vi "API.vi"() -> ()   [LabVIEW 2018]
uses:
  <vilib>/NI Veristand/Execution/Project/NI_VS Project ExecutionAPI.lvlib
  <vilib>/NI Veristand/Execution/Workspace/NI_VS Workspace ExecutionAPI.lvlib
  <vilib>/NI Veristand/Execution/ModelManager/NI_VS ModelManager ExecutionAPI.lvlib
  <vilib>/NI Veristand/Execution/Workspace/NI VeriStand - Get Multiple Channel Values.vi
  <vilib>/NI Veristand/Execution/ModelManager/NI VeriStand - Get Multiple Parameter Values.vi
  <vilib>/NI Veristand/Execution/ModelManager/NI VeriStand - Set Multiple Parameter Values.vi
  <vilib>/NI Veristand/Execution/DataLogging/NI_VS Data Logging API.lvlib
  <vilib>/NI Veristand/Execution/DataLogging/New Data Logging Specification (Text).vi
  <vilib>/NI Veristand/Execution/DataLogging/Text Channel.ctl
panel:
  in  "Channel Paths":T1[](array[typedef])
  in  "Session Name in":string="datalog"
  in  "Zapsat":bool
  out "Parametrz view":dbl[](array[numeric])
  in  "Parametry SET":dbl[](array[numeric])
  out "Aliases":string[](array[string])
  out "Parameters":string[](array[string])
  out "Values":dbl[](array[numeric])
  out "error out":errorcluster
  out "Channels":string[](array[string])
  in  "Project File Path":path=path "C:/Users/Public/Documents/National Instruments/NI VeriStand 2018/Projects/Example/Sinewave Delay.nivsproj"
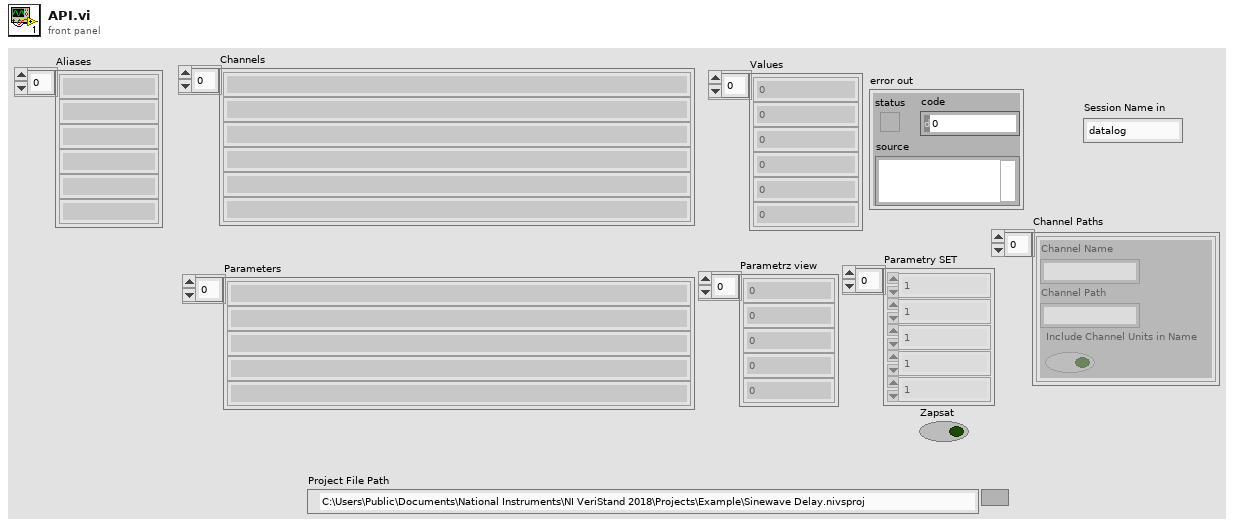
[diagram p1: front panel]
types:
  T1 = typedef "NI_VS Data Logging API.lvlib/Text Channel.ctl" = cluster{"Channel Name":string, "Channel Path":string, "Include Channel Units in Name":bool}
  T2 = typedef "NI_VS Project ExecutionAPI.lvlib/Project Ref.ctl" = refnum<k24>
  T3 = typedef "NI_VS Workspace ExecutionAPI.lvlib/WorkspaceAPI.ctl" = refnum<k24>
  T4 = typedef "NI_VS ModelManager ExecutionAPI.lvlib/ModelManagerAPI.ctl" = refnum<k24>
  T5 = typedef "NI_VS Data Logging API.lvlib/DataLoggingSpecification Ref.ctl" = refnum<k24>
  T6 = typedef "NI_VS Data Logging API.lvlib/IDataLogging Ref.ctl" = refnum<k24>
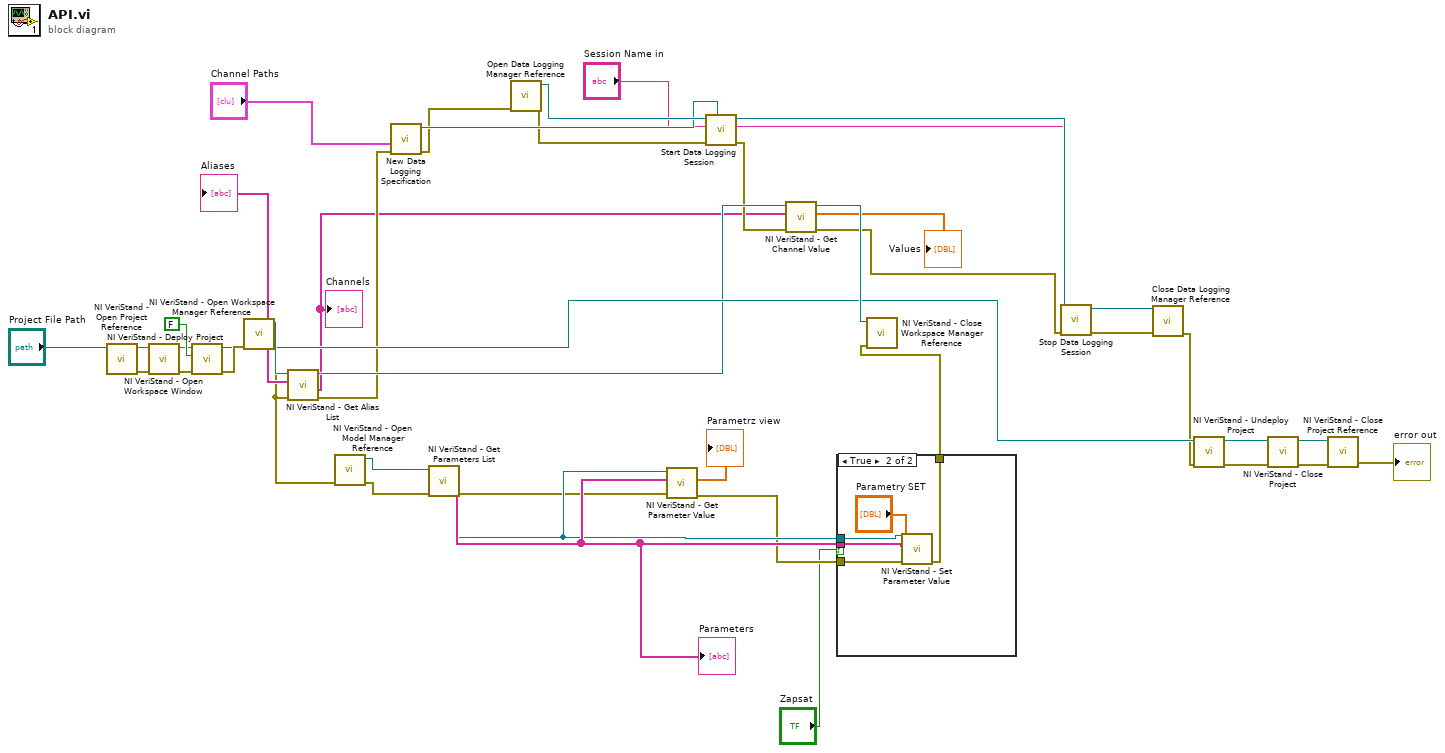
[diagram p0: block diagram]
diagram:
  n1 = call <vilib>:"NI VeriStand - Open Project Reference.vi"("Project File Path"="Project File Path") -> ("error out"=w40:errorcluster, "Project Ref"=w43:T2)  [unwired: 9 in]
  n2 = call <vilib>:"NI VeriStand - Open Workspace Window.vi"("error in (no error)"=w40, "Project Ref in"=w43) -> ("error out"=w39:errorcluster, "Project Ref out"=w35:T2)  [unwired: 8 in]
  n3 = call <vilib>:"NI VeriStand - Deploy Project.vi"("error in (no error)"=w39, "Show Progress (F)"=FALSE, "Project Ref in"=w35) -> ("error out"=w38:errorcluster, "Project Ref out"=w29:T2)  [unwired: 7 in]
  n4 = call <vilib>:"NI VeriStand - Open Workspace Manager Reference.vi"("error in (no error)"=w38) -> ("error out"=w23:errorcluster, "WorkspaceManager"=w36:T3)  [unwired: 9 in]
  n5 = call <vilib>:"NI VeriStand - Get Alias List.vi"("error in (no error)"=w23, "WorkspaceManager in"=w36) -> ("error out"=w7:errorcluster, "Channels"=w2:string[], "Aliases"=→"Aliases":string[], "WorkspaceManager out"=w27:T3)  [unwired: 6 in]
  "Channels" <- w2
  n6 = call <vilib>:"NI VeriStand - Open Model Manager Reference.vi"("error in (no error)"=w23) -> ("error out"=w24:errorcluster, "ModelManager"=w26:T4)  [unwired: 9 in]
  n7 = call-poly <vilib>:"New Data Logging Specification.vi"("error in (no error)"=w7, "Channel Paths"="Channel Paths") -> ("error out"=w6:errorcluster, "Data Logging Specification Ref out"=w12:T5)  [unwired: 8 in]
  n8 = call <vilib>:"NI VeriStand - Get Parameters List.vi"("error in (no error)"=w24, "ModelManager in"=w26) -> ("error out"=w19:errorcluster, "Parameters"=w22:string[], "ModelManager out"=w21:T4)  [unwired: 7 in]
  "Parameters" <- w22
  n9 = call <vilib>:"Open Data Logging Manager Reference.vi"("error in (no error)"=w6) -> ("error out"=w5:errorcluster, "Data Logging Manager Ref out"=w15:T6)  [unwired: 9 in]
  n10 = call-poly <vilib>:"NI VeriStand - Get Parameter Value.vi"("error in (no error)"=w19, "Parameters"=w22, "ModelManager in"=w21) -> ("error out"=w18:errorcluster, "Values"=→"Parametrz view":dbl[])  [unwired: 6 in, 1 out]
  n11 = call <vilib>:"Start Data Logging Session.vi"("Data Logging Specification Ref in"=w12, "error in (no error)"=w5, "Session Name in"="Session Name in", "Data Logging Manager Ref in"=w15) -> ("error out"=w4:errorcluster, "Session Name out"=w11:string, "Data Logging Manager Ref out"=w14:T6)  [unwired: 5 in]
  n12 = call-poly <vilib>:"NI VeriStand - Get Channel Value.vi"("error in (no error)"=w4, "Channels"=w2, "WorkspaceManager in"=w27) -> ("error out"=w3:errorcluster, "Values"=→"Values":dbl[], "WorkspaceManager out"=w30:T3)  [unwired: 6 in]
  n13 = case shown="True" "Zapsat" {
    tunnel: w22 -> [_ w48]
    tunnel: w21 -> [_ w47]
    tunnel: w18 -> [w44 w46]
    tunnel: [w44 w45] -> w17
    frame False {
    }
    frame True {
      n14 = call-poly <vilib>:"NI VeriStand - Set Parameter Value.vi"("error in (no error)"=w46, "Values"="Parametry SET", "Parameters"=w48, "ModelManager in"=w47) -> ("error out"=w45:errorcluster)  [unwired: 6 in, 1 out]
    }
  }
  n15 = call <vilib>:"NI VeriStand - Close Workspace Manager Reference.vi"("error in (no error)"=w17, "WorkspaceManager"=w30) -> ()  [unwired: 9 in, 1 out]
  n16 = call <vilib>:"Stop Data Logging Session.vi"("error in (no error)"=w3, "Session Name in"=w11, "Data Logging Manager Ref in"=w14) -> ("error out"=w9:errorcluster, "Data Logging Manager Ref out"=w13:T6)  [unwired: 5 in, 2 out]
  n17 = call <vilib>:"Close Data Logging Manager Reference.vi"("error in (no error)"=w9, "Data Logging Manager Ref in"=w13) -> ("error out"=w8:errorcluster)  [unwired: 9 in]
  n18 = call <vilib>:"NI VeriStand - Undeploy Project.vi"("error in (no error)"=w8, "Project Ref in"=w29) -> ("error out"=w33:errorcluster, "Project Ref out"=w32:T2)  [unwired: 8 in]
  n19 = call <vilib>:"NI VeriStand - Close Project.vi"("error in (no error)"=w33, "Project Ref in"=w32) -> ("error out"=w34:errorcluster, "Project Ref out"=w31:T2)  [unwired: 8 in]
  n20 = call <vilib>:"NI VeriStand - Close Project Reference.vi"("error in (no error)"=w34, "Project Ref"=w31) -> ("error out"=→"error out":errorcluster)  [unwired: 9 in]
